vi "Score Display - Load Image (LV).vi"(1 "path to image file":path) -> (0 "image data":T1)   [LabVIEW 2013]
uses:
  <vilib>/picture/picture.llb/imagedata.ctl
  Instance           4 39Saved   Score Display - Load Image (LV) .vi
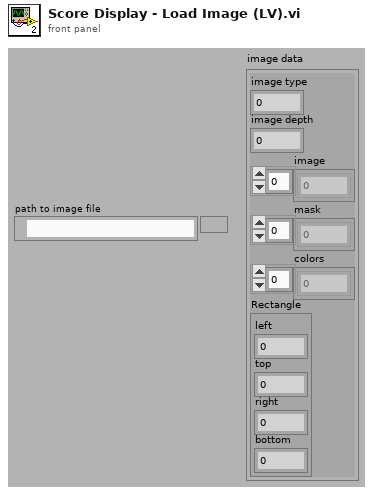
[diagram p1: front panel]
types:
  T1 = typedef "imagedata.ctl" = cluster{"image type":i32, "image depth":i32, "image":u8[], "mask":u8[], "colors":u32[], "Rectangle":cluster{"left":i16, "top":i16, "right":i16, "bottom":i16}}
  T2 = enum32{"invalid app kind", "Development System", "Run Time System", "Student Edition", "Embedded LabVIEW", "Evaluation", "Custom"}
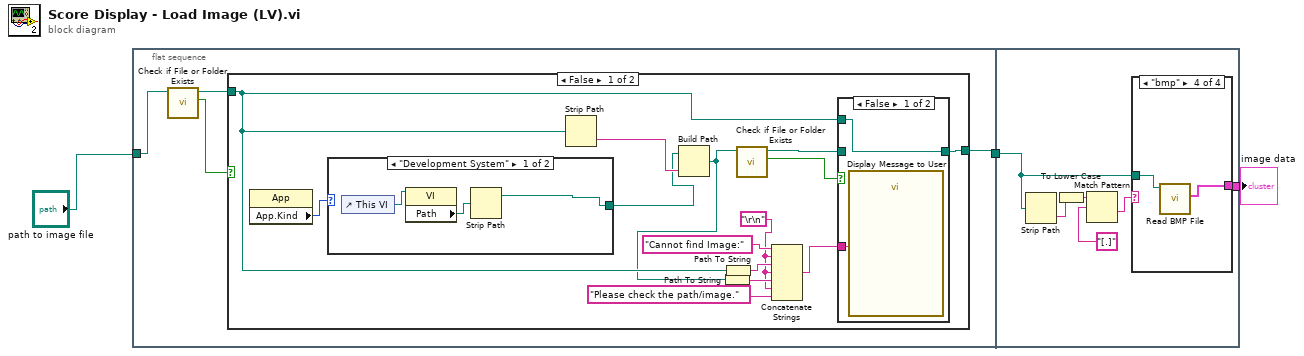
[diagram p0: block diagram]
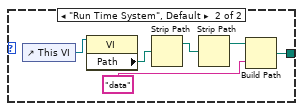
[diagram p2: hidden frame]
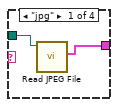
[diagram p5: hidden frame]
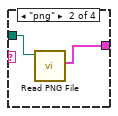
[diagram p6: hidden frame]
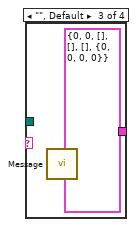
[diagram p7: hidden frame]
diagram:
  n1 = flat-sequence {
    tunnel: "path to image file" -> [w7]
    tunnel: [w4] -> w1
    tunnel: [w35] -> w2
    tunnel: w1 -> [w39]
    frame #0 {
      n2 = call <vilib>:"Check if File or Folder Exists.vi"("path"=w7) -> ("file or folder exists?"=w6:bool, "dup path"=w5:path)  [unwired: 8 in, 1 out]
      n3 = case shown="False" w6 {
        tunnel: [w19 w34] -> w4
        tunnel: w5 -> [w17 w34]
        frame False {
          w10 = "\r\n"
          n4 = property class="App"() -> ("App.Kind"=w8:T2)  [unwired: 2 in, 2 out]
          n5 = case shown="\"Development System\"" w8 {
            tunnel: [w22 w27] -> w9
            frame "Development System" {
              n6 = control-ref of="This VI"() -> (w24:refnum<vi>)
              n7 = property class="VI"(reference=w24) -> ("Path"=w23:path)  [unwired: 1 in, 2 out]
              n8 = Strip Path(path=w23) -> (stripped path=w22:path)  [unwired: 1 out]
            }
            frame "Run Time System", Default {
              n9 = control-ref of="This VI"() -> (w30:refnum<vi>)
              n10 = property class="VI"(reference=w30) -> ("Path"=w29:path)  [unwired: 1 in, 2 out]
              n11 = Strip Path(path=w29) -> (stripped path=w26:path)  [unwired: 1 out]
              n12 = Strip Path(path=w26) -> (stripped path=w25:path)  [unwired: 1 out]
              n13 = Build Path(base path=w25, name or relative path="data") -> (appended path=w27:path)
            }
          }
          n14 = Strip Path(path=w17) -> (name=w18:string)  [unwired: 1 out]
          n15 = Build Path(base path=w9, name or relative path=w18) -> (appended path=w13:path)
          n16 = Path To String(path=w13) -> (string=w11:string)
          n17 = Path To String(path=w17) -> (string=w16:string)
          n18 = call <vilib>:"Check if File or Folder Exists.vi"("path"=w13) -> ("file or folder exists?"=w21:bool, "dup path"=w20:path)  [unwired: 8 in, 1 out]
          n19 = Concatenate Strings("Cannot find Image:", w10, w16, w10, w11, w10, "Please check the path/image.") -> (w14:string)
          n20 = case shown="False" w21 {
            tunnel: w20 -> [_ w33]
            tunnel: [w31 w33] -> w19
            tunnel: w14 -> [w32 _]
            tunnel: w17 -> [w31 _]
            frame False {
              n21 = call "Display Message to User"("Message"=w32) -> ()  [unwired: 9 in, 2 out]
            }
            frame True {
            }
          }
        }
        frame True {
        }
      }
    }
    frame #1 {
      n22 = Strip Path(path=w39) -> (name=w37:string)  [unwired: 1 out]
      n23 = To Lower Case(string=w37) -> (all lower case string=w36:string)
      n24 = Match Pattern(string=w36, regular expression="[.]") -> (after substring=w38:string)  [unwired: 4 out]
      n25 = case shown="\"bmp\"" w38 {
        tunnel: w39 -> [w41 w44 _ w47]
        tunnel: [w42 w43 T1 {"image type"=0, "image depth"=0, "image"=[], "mask"=[], "colors"=[], "Rectangle"={"left"=0, "top"=0, "right"=0, "bottom"=0}} ("image data") w46] -> w35
        frame "jpg" {
          n26 = call <vilib>:"Read JPEG File.vi"("path to JPEG file"=w41) -> ("image data"=w42:T1)  [unwired: 1 in, 9 out]
        }
        frame "png" {
          n27 = call <vilib>:"Read PNG File.vi"("path to PNG file"=w44) -> ("image data"=w43:T1)  [unwired: 1 in, 9 out]
        }
        frame "", Default {
          n28 = call "Message"() -> ()  [unwired: 3 in, 9 out]
        }
        frame "bmp" {
          n29 = call <vilib>:"Read BMP File.vi"("path to BMP file"=w47) -> ("image data"=w46:T1)  [unwired: 1 in, 9 out]
        }
      }
    }
  }
  "image data" <- w2
